vi "DAT Example.vi"() -> ()   [LabVIEW 2016, in "LVtoITX.lvclass"]
uses:
  LVtoITX.lvclass
panel:
  out "data rows saved":i32
  in  "stop":bool
  in  "number4":dbl=7.0
  in  "number3":dbl=5.0
  in  "number2":dbl=3.0
  in  "number1":dbl
  in  "wavenames (.Vx, etc)":string[](array[string])=["time", "temp", "Bfield", "X0", "Y0", "X1", "Y1", "X2", "Y2", "X3", "Y3", "X4", "Y4", "X5", "Y5"]
  out "plot2":cluster{"X":dbl[], "Y":dbl[]}[](graph)
  out "plot1":cluster{"X":dbl[], "Y":dbl[]}[](graph)
  out "plot0":cluster{"X":dbl[], "Y":dbl[]}[](graph)
  in  "Notes":string="date and time are AUTOMATICALLY saved!\nwrite your experiment notes here"
  in  "path":path=path "C:/"
  in  "filename":string="datatest"
  # "- set path to folder\n- set base filename\n   (up to 999,999 files with same base name \n    an be written in one folder)\n- type some comments"
  # "you usually display your data as a XY\ngraphs or charts:"
  # "give everything you are saving a name,\nor else you will become confused!"
  # "initialize your file using the structure shown at right\n----------------->"
  # "wire the path using the output from the initialize step\n\ncombine all of your data using \"build  array\" function\n\nEach entry represents one data point at a partiular time"
  # "numbers can be\n saved too:"
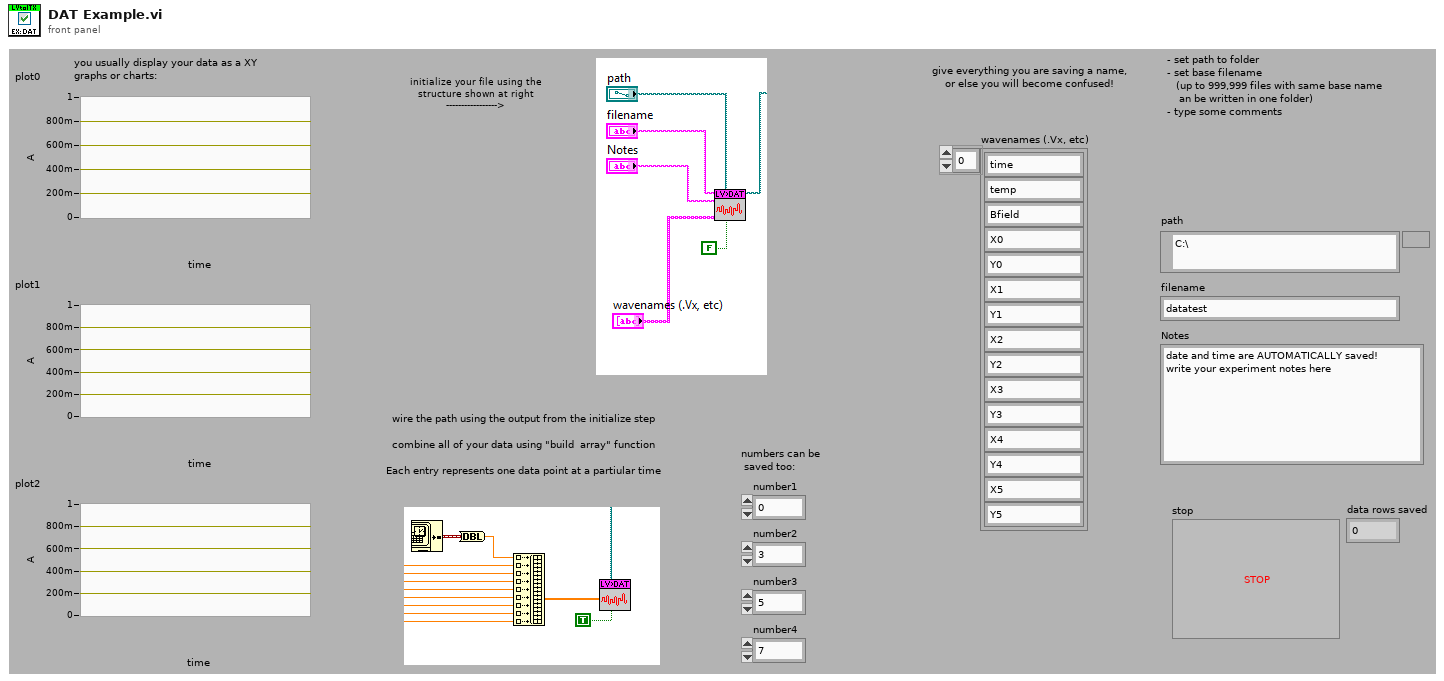
[diagram p1: front panel]
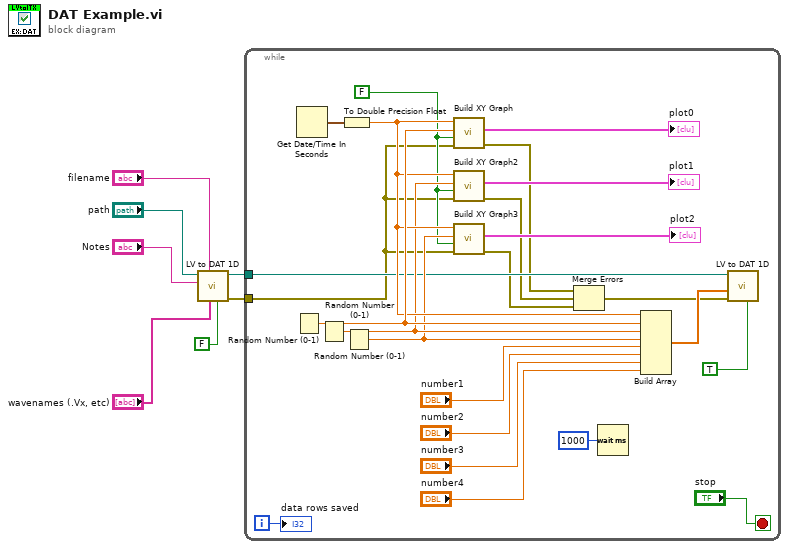
[diagram p0: block diagram]
diagram:
  n1 = call "LV to DAT 1D.vi"("append to file? (new file:F)"=FALSE, "wavenames (.Vx, etc)"="wavenames (.Vx, etc)", "filename"="filename", "Comments"="Notes", "path"="path") -> ("error out"=w7:errorcluster, "new file path"=w3:path)  [unwired: 5 in]
  n2 = while {
    tunnel: w3 -> [w13]
    tunnel: w7 -> [w12]
    i -> [w16]
    stop <- "stop" stop-if-true
    w19 = FALSE ("Reset")
    n3 = Random Number (0-1)() -> (number: 0 to 1=w26:dbl)
    n4 = Get Date/Time In Seconds() -> (seconds since 1Jan1904=w27:timestamp)
    n5 = Random Number (0-1)() -> (number: 0 to 1=w24:dbl)
    n6 = To Double Precision Float(number=w27) -> (double precision float=w25:dbl)
    n7 = Random Number (0-1)() -> (number: 0 to 1=w23:dbl)
    n8 = call "Build XY Graph"("error in (no error)"=w12, "Reset"=w19, "Y Input"=w26, "X Input"=w25) -> ("error out"=w11:errorcluster, "XY Graph"=→"plot0":cluster{"X":dbl[], "Y":dbl[]}[])  [unwired: 6 in]
    n9 = call "Build XY Graph2"("error in (no error)"=w12, "Reset"=w19, "Y Input"=w24, "X Input"=w25) -> ("error out"=w10:errorcluster, "XY Graph"=→"plot1":cluster{"X":dbl[], "Y":dbl[]}[])  [unwired: 6 in]
    n10 = call "Build XY Graph3"("error in (no error)"=w12, "Reset"=w19, "Y Input"=w23, "X Input"=w25) -> ("error out"=w9:errorcluster, "XY Graph"=→"plot2":cluster{"X":dbl[], "Y":dbl[]}[])  [unwired: 6 in]
    n11 = Merge Errors(w11, w10, w9) -> (w8:errorcluster)
    n12 = Wait (ms)(milliseconds to wait=u32 1000) -> ()  [unwired: 1 out]
    n13 = Build Array(w25, w26, w24, w23, "number1", "number2", "number3", "number4") -> (w14:dbl[])
    n14 = call "LV to DAT 1D.vi"("append to file? (new file:F)"=TRUE, "error in"=w8, "Data"=w14, "path"=w13) -> ()  [unwired: 6 in, 2 out]
    "data rows saved" <- w16
  }
